vi "test Log File.vi"(8 "error in":errorcluster, 11 "TestCase in":refnum<class "Embedded Data Logger System Tests.lvclass">) -> (0 "error out":errorcluster, 3 "TestCase out":refnum<class "Embedded Data Logger System Tests.lvclass">)   [LabVIEW 2018, in "Embedded Data Logger System Tests.lvclass"]
uses:
  Embedded Data Logger System Tests.lvclass
  <vilib>/addons/_JKI Toolkits/VI Tester/TestCase.llb/TestCase.lvclass
  C:/Program Files (x86)/National Instruments/LabVIEW 2018/vi.lib/addons/_JKI Toolkits/VI Tester/TestCase.llb/TestCase.lvclass
panel:
  out "End Time":dbl
  out "Start Time":dbl
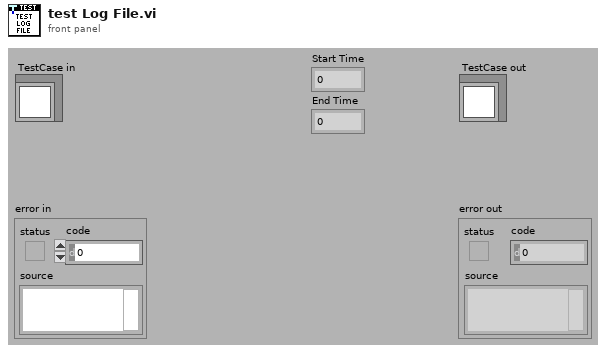
[diagram p1: front panel]
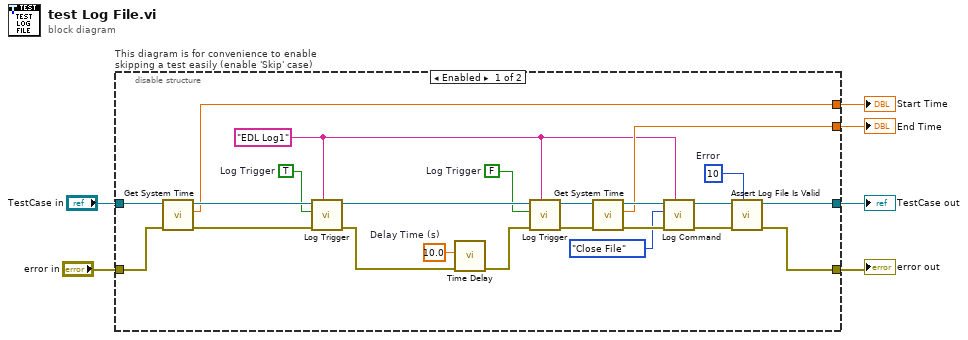
[diagram p0: block diagram]
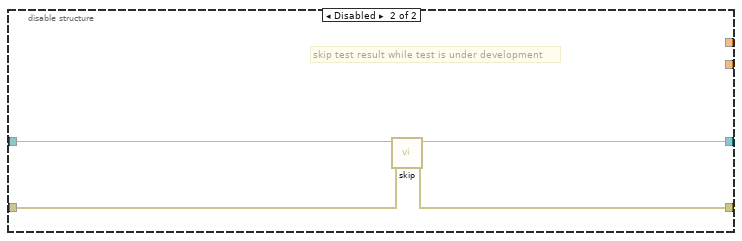
[diagram p2: hidden frame]
diagram:
  n1 = disable-structure "This diagram is for convenience to enable skipping a test easily (enable 'Skip' case)" shown="Enabled" {
    disable-tunnel: "TestCase in" -> [w29 w33]
    disable-tunnel: [w13 w31] -> w3
    disable-tunnel: [w12 w32] -> w5
    disable-tunnel: "error in" -> [w28 w30]
    disable-tunnel: [w9 _] -> w2
    disable-tunnel: [w8 _] -> w1
    frame Enabled {
      w7 = "EDL Log1" ("Embedded Data Logger File Name")
      w10 = 10  # Error
      w19 = FALSE  # Log Trigger
      w20 = 10.0  # Delay Time (s)
      w23 = TRUE  # Log Trigger
      n2 = call "Get System Time.vi"("error in (no error)"=w28, "Embedded Data Logger System Tests in"=w29) -> ("error out"=w26:errorcluster, "System Time"=w8:dbl, "Embedded Data Logger System Tests out"=w27:refnum<class "Embedded Data Logger System Tests.lvclass">)  [unwired: 7 in]
      n3 = call "Log Trigger.vi"("Embedded Data Logger File Name"=w7, "error in"=w26, "Log Trigger"=w23, "Embedded Data Logger System Tests in"=w27) -> ("error out"=w24:errorcluster, "Embedded Data Logger System Tests out"=w25:refnum<class "Embedded Data Logger System Tests.lvclass">)  [unwired: 6 in]
      n4 = call "Time Delay"("error in (no error)"=w24, "Delay Time (s)"=w20) -> ("error out"=w21:errorcluster)  [unwired: 9 in]
      n5 = call "Log Trigger.vi"("Embedded Data Logger File Name"=w7, "error in"=w21, "Log Trigger"=w19, "Embedded Data Logger System Tests in"=w25) -> ("error out"=w17:errorcluster, "Embedded Data Logger System Tests out"=w22:refnum<class "Embedded Data Logger System Tests.lvclass">)  [unwired: 6 in]
      n6 = call "Get System Time.vi"("error in (no error)"=w17, "Embedded Data Logger System Tests in"=w22) -> ("error out"=w15:errorcluster, "System Time"=w9:dbl, "Embedded Data Logger System Tests out"=w18:refnum<class "Embedded Data Logger System Tests.lvclass">)  [unwired: 7 in]
      n7 = call "Log Command.vi"("Embedded Data Logger File Name"=w7, "error in"=w15, "Log Command"=enum16{"Idle", "Open File", "Close File"}."Close File", "Embedded Data Logger System Tests in"=w18) -> ("error out"=w11:errorcluster, "Embedded Data Logger System Tests out"=w16:refnum<class "Embedded Data Logger System Tests.lvclass">)  [unwired: 6 in]
      n8 = call "Assert Log File Is Valid.vi"("Error"=w10, "error in (no error)"=w11, "Embedded Data Logger System Tests in"=w16) -> ("error out"=w12:errorcluster, "Embedded Data Logger System Tests out"=w13:refnum<class "Embedded Data Logger System Tests.lvclass">)  [unwired: 7 in]
    }
    frame Disabled {
      # "skip test result while test is under development"
      n9 = call <vilib>:"skip.vi"("error in (no error)"=w30, "TestCase in"=w33) -> ("error out"=w32:errorcluster, "TestCase out"=w31:refnum<class "Embedded Data Logger System Tests.lvclass">)  [unwired: 8 in]
    }
  }
  "error out" <- w5
  "TestCase out" <- w3
  "Start Time" <- w1
  "End Time" <- w2
